vi "OCT ATS660.vi"() -> ()   [LabVIEW 2014]
doc: "I. Description:\nThis example demonstrates how to acquire a continuous amount of data (Waveform) using the DAQ device's internal clock.\n\nII. Instructions for Running:\n1. Create an analog input voltage channel.\n2. Set the rate for the sample clock. Additionally, define the sample mode to be continuous.\n3. Call the Start VI to start the acquisition.\n4. Read the waveform data in a loop until the user hits the stop button or an error occurs.\nNote: This example reads data from one or more channels and returns an array of data. Use the Index Array function to access an individual channel of data.\n5. Call the Clear Task VI to clear the Task.\n6. Use the popup dialog box to display an error if any.\n\nIV. I/O Connections Overview:\nMake sure your signal input terminal matches the Physical Channel I/O Control. For further connection information, refer to your hardware reference manual."
uses:
  Type Defs/OCT DAQ Channel Data Type.ctl
  Type Defs/Display States.ctl
  Saving Data/Saving Data States.ctl
  Type Defs/OCT Hardware States.ctl
  Type Defs/OCT Imaging Parameters Cluster.ctl
  Alazar VIs/ATS_ctl/ATS_Async_Setting.ctl
  Galvo VIs/galvo_states.ctl
  Alazar VIs/ATS_ctl/ATS_Global.ctl
  Alazar VIs/ATS_ctl/Record.ctl
  Alazar VIs/ATS_ctl/Clock.ctl
  Alazar VIs/ATS_ctl/ClockSource.ctl
  Alazar VIs/ATS_ctl/ClockRate.ctl
  Alazar VIs/ATS_ctl/ClockEdge.ctl
  Alazar VIs/ATS_ctl/InputCtrl.ctl
  Alazar VIs/ATS_ctl/Coupling.ctl
  Alazar VIs/ATS_ctl/Range.ctl
  Alazar VIs/ATS_ctl/Impedance.ctl
  Alazar VIs/ATS_ctl/Bandwidth.ctl
  Alazar VIs/ATS_ctl/Trigger.ctl
  Alazar VIs/ATS_ctl/TriggerOperation.ctl
  Alazar VIs/ATS_ctl/TriggerEngine.ctl
  Alazar VIs/ATS_ctl/ExtTrigger.ctl
  Alazar VIs/ATS_ctl/ExtTrigRange.ctl
  Signal Processing/processing_states.ctl
  En Face/En Face Depth Parameters.ctl
  Alazar VIs/ATS_ctl/ATS_Async_Ctrl.ctl
  Alazar VIs/ATS_ctl/ATS_Async_Mode.ctl
  Alazar VIs/ATS_ctl/ATS_DMA_Channel.ctl
  Alazar VIs/ATS_ctl/ATS_ReadSamples.ctl
  Alazar VIs/ATS_ctl/Device_Ctrl.ctl
  Alazar VIs/ATS_ctl/ATS_Check_Ctrl.ctl
  En Face/En Face States.ctl
  DAQ Status States.ctl
  Signal Processing/Display Raw Data states.ctl
panel:
  out "Background Array":u16[](array[numeric])
  in  "Calibrate":bool
  in  "Save Sweep Button":bool
  in  "Linear?":bool
  in  "Data Format":T1
  out "BScan":sgl[][](graph)
  in  "Display":T2
  in  "Save Sweep":bool
  in  "Stop Button":bool
  out "B-Scans Per Buffer":i32=1
  out "Current State":T3=enum."Aquire and Save"
  in  "Channels":tag="Dev2/ao0:1"
  in  "Trigger Source":tag="/Dev2/PFI7"
  in  "Imaging Parameters":T4={"Points Per A-Scan"=0, "A-Scans per B-Scan"=0, "Voltage Range"=1.0, "Card Resolution (bits)"=12}
  out "First Time?":bool=TRUE
  out "Save Data":bool
  in  "Async_Setting":T5
  out "Processing Finished":bool
  in  "OCT Hardware States":T3=enum."Acquire Clock"
  out "Save State":T6=enum."Do Nothing"
  out "Clock Length":u32=9184
  out "Reset DAQ":bool
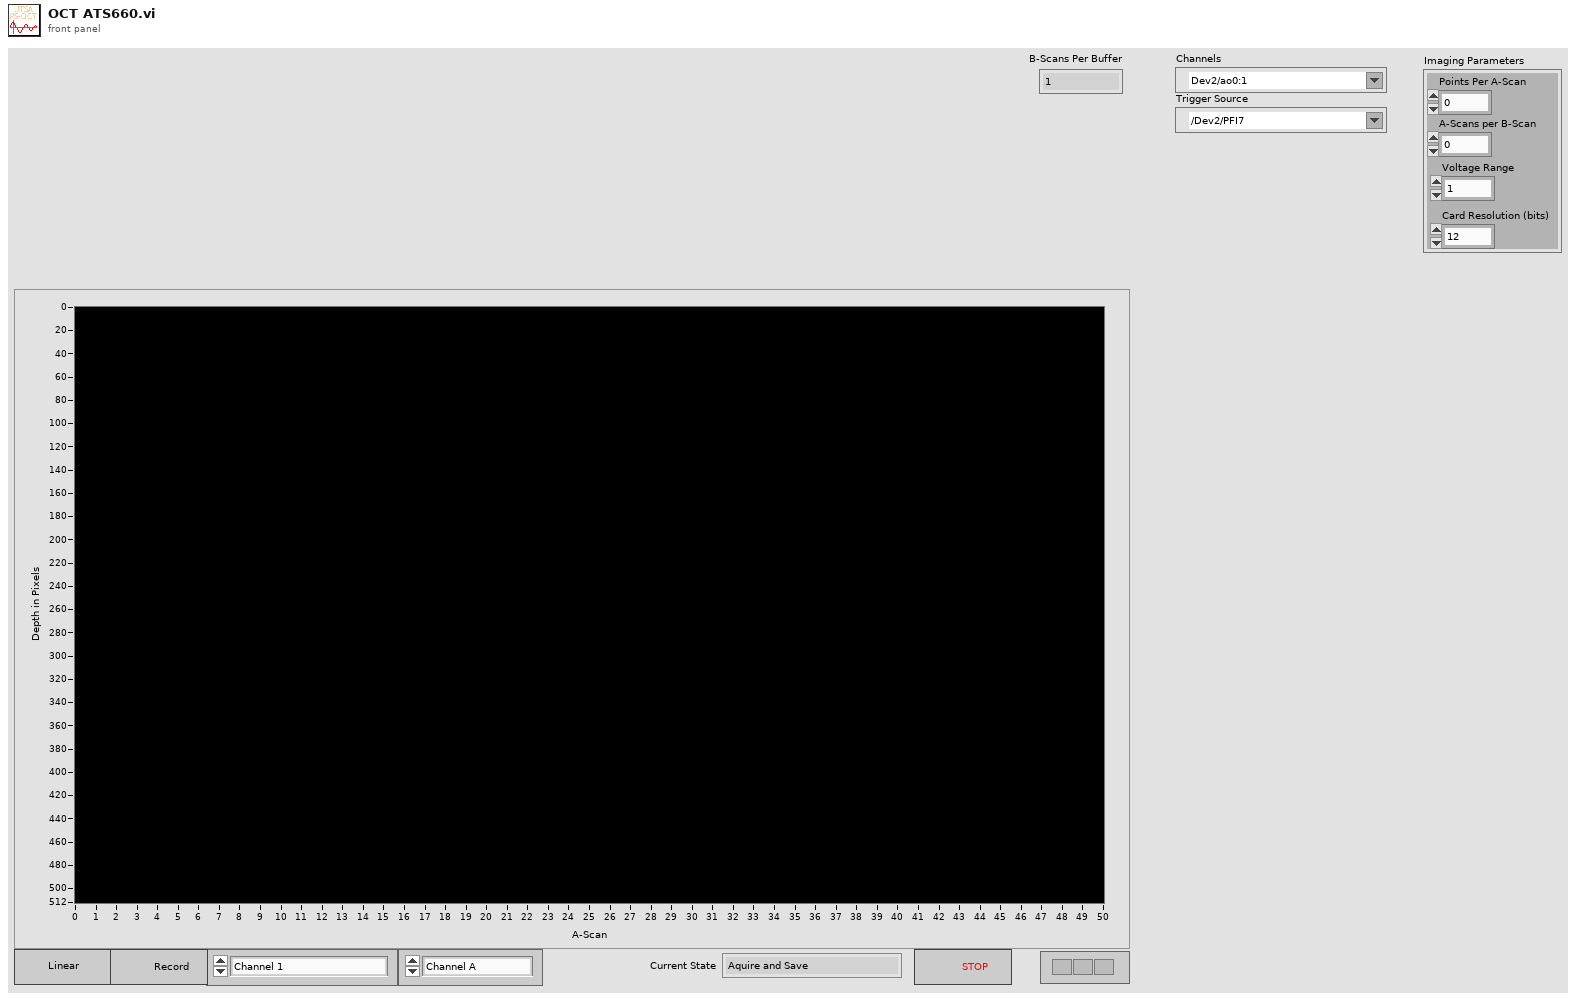
[diagram p1: front panel]
types:
  T1 = typedef "OCT DAQ Channel Data Type.ctl" = enum16{"Channel 1", "Channel 2", "Channel 1 and 2"}
  T2 = typedef "Display States.ctl" = enum16{"Channel A", "Channel B"}
  T3 = typedef "OCT Hardware States.ctl" = enum16{"Acquire Data", "Aquire and Save", "Allocate OpenCL Memory", "Delete OpenCL Memory", "Background Subtraction", "Acquire Background", "K-Space Calibration", "Update DAQ Parameters", "Initialize Clock", "Stop", "Wait", "Acquire Clock", "Initialize DAQ", "Set Resampling Array"}
  T4 = typedef "OCT Imaging Parameters Cluster.ctl" = cluster{"Points Per A-Scan":i32, "A-Scans per B-Scan":i32, "Voltage Range":sgl, "Card Resolution (bits)":u16}
  T5 = typedef "ATS_Async_Setting.ctl" = cluster{"UseHeader":u32, "Rec/Buffer":u32, "Total_Rec":u32, "DataBuffer":bool, "GetProcessedData":bool}
  T6 = typedef "Saving Data States.ctl" = enum16{"Get Queue Size", "Get Queue", "Get Timeout", "Flush Queue", "Close Files", "Create Files", "Do Nothing", "Initialize", "Enqueue Data", "Save Data", "Shutdown"}
  T7 = typedef "ATS_Global.ctl" = cluster{"Record":T8, "Clock":T9, "Input A":T13, "Input B":T13, "Trigger":T18}
  T8 = typedef "Record.ctl" = cluster{"Count":u32, "Presize":u32, "Length":u32}
  T9 = typedef "Clock.ctl" = cluster{"ClckSource":T10, "ClckRate":T11, "ClckEdge":T12, "Decimation":u32}
  T10 = typedef "ClockSource.ctl" = enum16{"Internal", "External", "Medium Ext.", "Slow Ext.", "Ext. AC", "Ext. DC", "Ext. (PLL)"}
  T11 = typedef "ClockRate.ctl" = u32
  T12 = typedef "ClockEdge.ctl" = u16
  T13 = typedef "InputCtrl.ctl" = cluster{"Coupling":T14, "Range":T15, "Impedance":T16, "Bandwidth":T17}
  T14 = typedef "Coupling.ctl" = enum16{"AC", "DC"}
  T15 = typedef "Range.ctl" = u32
  T16 = typedef "Impedance.ctl" = enum16{"1M ohms", "50 ohms"}
  T17 = typedef "Bandwidth.ctl" = enum16{"Full Bandwidth", "Reduce Bandwidth"}
  T18 = typedef "Trigger.ctl" = cluster{"TrigOperation":T19, "Timeout (s)":dbl, "Trig. Delay":u32, "Engine X":T20, "Engine Y":T20, "ExtTrigControl":T21}
  T19 = typedef "TriggerOperation.ctl" = enum16{"Only X", "Only Y", "X or Y", "X and Y", "X xor Y", "X and not Y", "not X and Y"}
  T20 = typedef "TriggerEngine.ctl" = cluster{"Source":enum32{"Chan_A", "Chan_B", "External", "Disable"}, "Slope":enum32{"Positive", "Negative"}, "Level":u32}
  T21 = typedef "ExtTrigger.ctl" = cluster{"Coupling":T14, "Range":T22}
  T22 = typedef "ExtTrigRange.ctl" = enum16{"1 V", "5 V", "TTL"}
  T23 = typedef "galvo_states.ctl" = enum16{"Reset", "Reset Galvos?", "Center Galvos", "Register Callback", "Get Scan Parameters", "Show", "Initialize", "Run Raster", "Load Raster", "Run Circle", "Shutdown"}
  T24 = typedef "processing_states.ctl" = enum16{"Initialize", "Set Background", "Update Imaging Parameters", "Get Queue", "Process Data", "Get Size", "Flush Data", "Set Reample Array", "Get Last Processed BScan", "Shutdown"}
  T25 = typedef "En Face Depth Parameters.ctl" = cluster{"En Face Start\nDepth":i32, "En Face End\nDepth":i32}
  T26 = typedef "En Face States.ctl" = enum16{"Save BMP", "Show", "Clear En Face", "Update EnFace"}
  T27 = typedef "Scanning Cluster.ctl" = cluster{"Fast Axis Offset":sgl, "Slow Axis Offset":sgl, "Slow Axis Amp":sgl, "Fast Axis Amp":sgl, "B-scans (rings)":u32, "A(cluster)/B":u32, "Scan Pattern":enum16{"Raster"}}
  T28 = typedef "Processed OCT Data.ctl" = cluster{"Intensity A":sgl[][][], "Intensity B":sgl[][][]}
  T29 = typedef "ATS_Async_Ctrl.ctl" = enum16{"SetupDMA", "StartCapture", "Get", "Get_Stream", "Abort", "Stop"}
  T30 = typedef "ATS_ReadSamples.ctl" = cluster{"Offset":i32, "Length":u32}
  T31 = typedef "ATS_DMA_Channel.ctl" = enum16{"Channel_A", "Channel_B", "A & B"}
  T32 = typedef "ATS_Async_Mode.ctl" = enum16{"Continuous", "Triggered", "No-Pre-Trigger", "Traditional"}
  T33 = typedef "ATS_Check_Ctrl.ctl" = enum16{"None", "NO_ATS9462", "ATS9462_Traditional", "Verify Board", "OnBoard Memory", "Board & Memory", "Master/Slave", "NO Master/Slave"}
  T34 = typedef "Device_Ctrl.ctl" = enum16{"Status", "About", "Arm", "ForceTrig", "Abort", "Initialize", "Init (NoPreset)", "Info", "Close", "Calibrate", "SetManually", "LED_ON", "LED_OFF"}
  T35 = typedef "DAQ Status States.ctl" = enum16{"Get", "Show"}
  T36 = typedef "ATS_Async_Status.ctl" = cluster{"Start DMA":bool, "StartCapture":bool, "Valid":bool, "Completed":bool, "InProgress":bool, "Timeout":bool, "Overflow":bool, "Error":bool}
  T37 = typedef "Display Raw Data states.ctl" = enum16{"Add Raw", "Add Processed", "Show"}
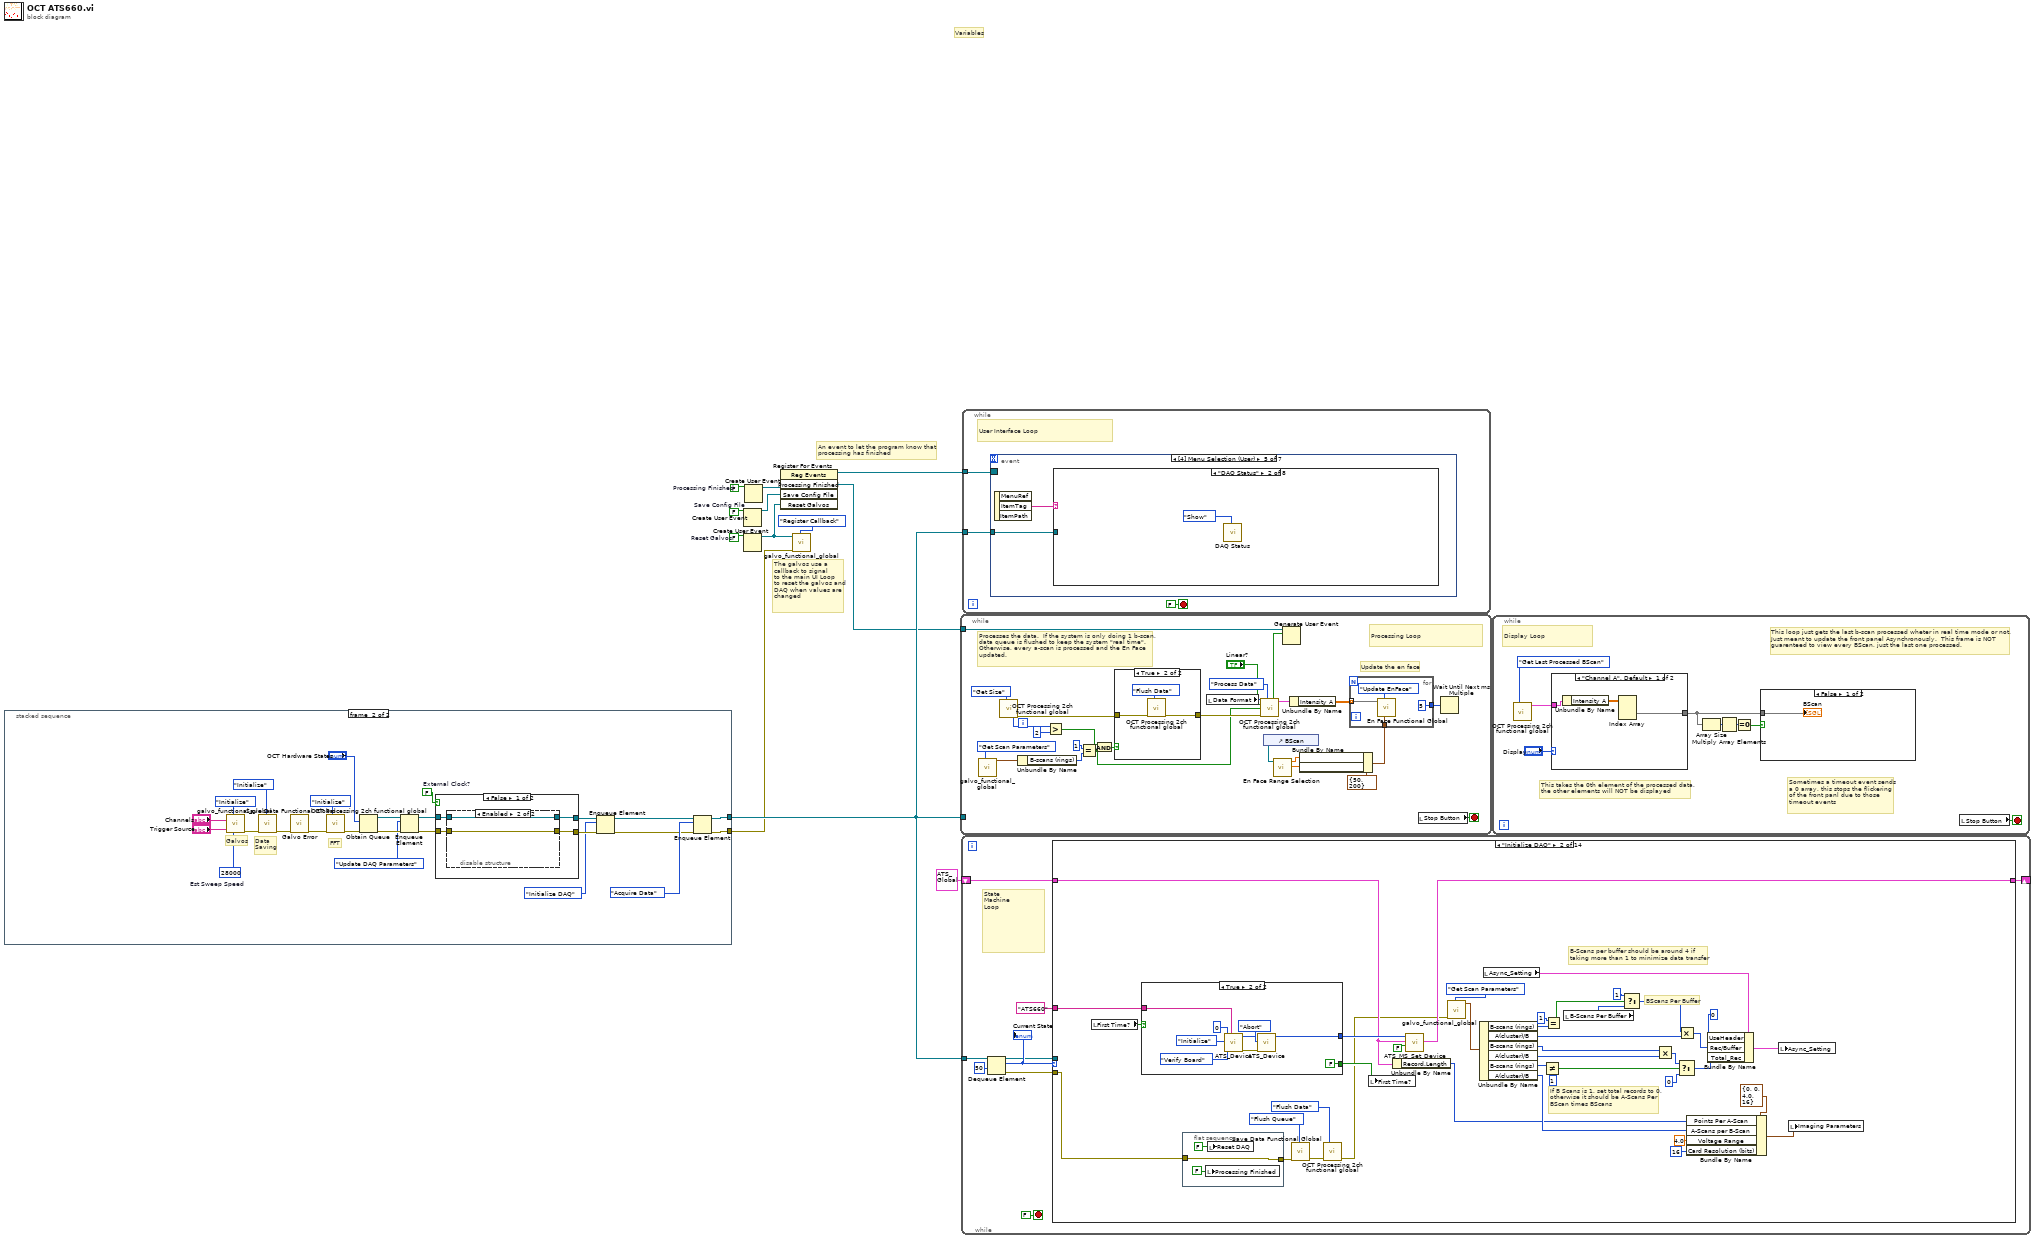
[diagram p0: block diagram]
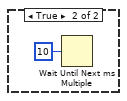
[diagram p3: hidden frame]
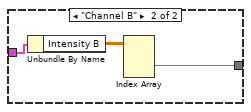
[diagram p4: hidden frame]
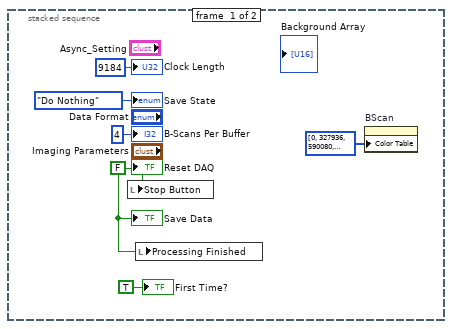
[diagram p5: hidden frame]
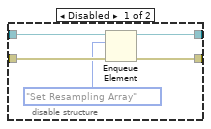
[diagram p6: hidden frame]
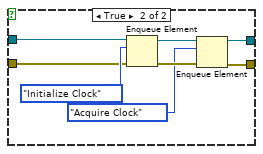
[diagram p7: hidden frame]
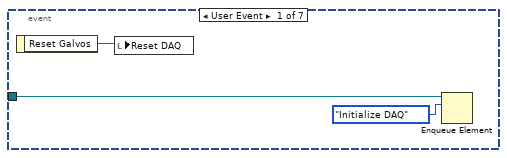
[diagram p8: hidden frame]
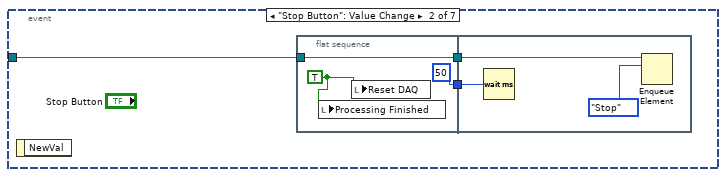
[diagram p9: hidden frame]
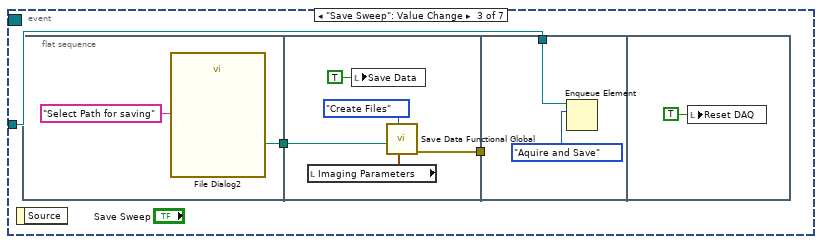
[diagram p10: hidden frame]
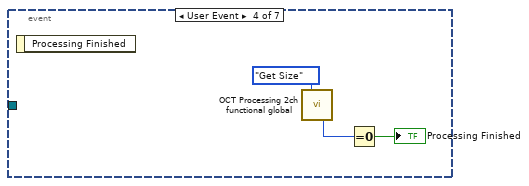
[diagram p11: hidden frame]
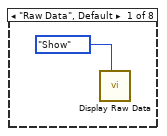
[diagram p12: hidden frame]
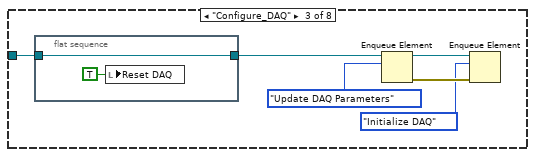
[diagram p13: hidden frame]
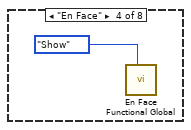
[diagram p14: hidden frame]
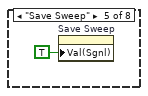
[diagram p15: hidden frame]
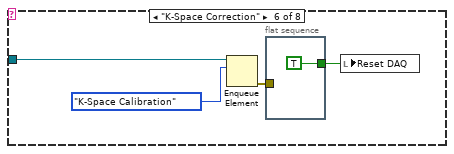
[diagram p16: hidden frame]
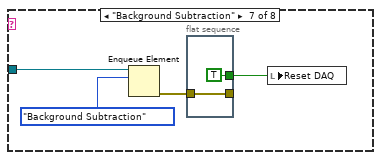
[diagram p17: hidden frame]
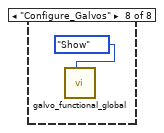
[diagram p18: hidden frame]
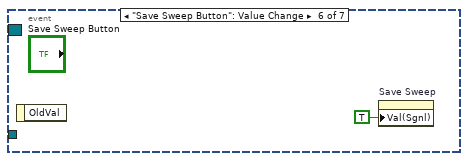
[diagram p19: hidden frame]
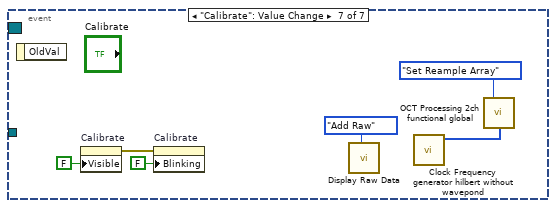
[diagram p20: hidden frame]
diagram:
  w5 = FALSE  # Reset Galvos
  w8 = FALSE  # Save Config File
  w11 = FALSE  # Processing Finished
  # "The galvos use a \ncallback to signal\nto the main UI Loop\nto reset the galvos and\nDAQ when values are\nchanged"
  # "An event to let the program know that\nprocessing has finished"
  # "Variables"
  n1 = stacked-sequence {
    tunnel: [_ w26] -> w9
    tunnel: [_ w25] -> w1
    frame #0 {
      w14 = FALSE ("Sweep Ready for saving")
      n2 = local write "Stop Button"(w14) -> ()
      n3 = local write "Processing Finished"(w14) -> ()
      n4 = property on="BScan" class="IntGraph (strict)"("Color Table"=u32[] [0, 327936, 590080, 852224, 983296, 1114624, 1180160, 1311232, 1442304, 1573632, 1704704, 1770240, 1901312, 1966848, 2098176, 2163712, 2294784, 2491392, 2557184, 2688256, 2753792, 2884864, 2950656, 3081728, 3147264, 3344129, 3475457, 3540993, 3672321, 3738113, 3869185, 3934977, 4066305, 4197633, 4328961, 4394497, 4460289, 4591617, 4657409, 4788481, 4854273, 4985601, 5116929, 5248257, 5314049, 5379841, 5511169, 5576961, 5708033, 5773825, 5905153, 6036482, 6167810, 6233346, 6299138, 6430466, 6496258, 6562050, 6693634, 6759426, 6890754, 7022082, 7087874, 7153666, 7284994, 7350786, 7482114, 7547906, 7613698, 7745026, 7876354, 8007682, 8073474, 8139522, 8205314, 8336642, 8467970, 8533763, 8599555, 8665347, 8731139, 8862467, 8993795, 9059587, 9125380, 9191428, 9257220, 9388548, 9454340, 9520132, 9585924, 9717253, 9848837, 9914629, 9980165, 10045957, 10177541, 10243334, 10309126, 10375174, 10440966, 10572294, 10703623, 10769416, 10835208, 10901256, 10967049, 11033097, 11033609, 11099401, 11165450, 11231242, 11231754, 11297547, 11363339, 11429131, 11495180, 11495692, 11561740, 11693069, 11758861, 11759373, 11825165, 11891214, 11957006, 12022799, 12023311, 12089103, 12220944, 12286736, 12286736, 12352529, 12418577, 12484370, 12550162, 12615954, 12681747, 12747796, 12813588, 12813845, 12879894, 12945686, 13077015, 13142808, 13143064, 13208856, 13274905, 13340697, 13340953, 13472282, 13538075, 13604379, 13670172, 13735964, 13801757, 13867550, 13933343, 13999392, 13999648, 14065441, 14131234, 14197027, 14197541, 14263334, 14329383, 14395176, 14460969, 14592553, 14658346, 14724139, 14789932, 14790189, 14856238, 14922287, 14988080, 15053873, 15054130, 15119923, 15185972, 15251765, 15317559, 15383353, 15449146, 15449660, 15515454, 15515968, 15516226, 15582021, 15582278, 15582536, 15648587, 15648844, 15714639, 15714897, 15715155, 15780949, 15781463, 15847256, 15847770, 15848028, 15913823, 15914081, 15979875, 15980133, 15980391, 16046441, 16046444, 16046703, 16046705, 16112500, 16113015, 16113274, 16113277, 16179072, 16179330, 16179588, 16245384, 16245387, 16245389, 16245648, 16311443, 16376982, 16377241, 16377499, 16443294, 16443553, 16443555, 16443815, 16509866, 16510124, 16510127, 16575923, 16575924, 16576182, 16576441, 16576443, 16576702, 16576705, 16576963, 16577222, 16577224, 16577482, 16577485, 16577743, 16577745, 16578004, 16578262, 16578264, 16578523, 16578782, 16579040, 16579299, 16579301, 16579303, 16579562, 16579821]) -> ()  [unwired: 2 in, 2 out]
      "B-Scans Per Buffer" <- 4 ("B-Scans Per Buffer")
      "Clock Length" <- u32 9184 ("Clock Length")
      "Save State" <- Saving_Data_States."Do Nothing" ("Save State")
      "Reset DAQ" <- w14
      "Save Data" <- w14
      "First Time?" <- TRUE ("First Time?")
    }
    frame #1 {
      w30 = 28000  # Est Sweep Speed
      w31 = FALSE  # External Clock?
      # "FFT"
      # "Data \nSaving"
      # "Galvos"
      n5 = call "galvo_functional_global.vi"("Est Sweep Speed"=w30, "State"=galvo_states."Initialize", "Trigger Source"="Trigger Source", "Analog Output"="Channels") -> ("error out"=w35:errorcluster)  [unwired: 6 in, 1 out]
      n6 = call "Save Data Functional Global.vi"("States"=Saving_Data_States."Initialize", "error in (no error)"=w35) -> ("error out"=w21:errorcluster)  [unwired: 6 in, 3 out]
      n7 = call "Galvo Error.vi"("error in (no error)"=w21) -> ("error out"=w20:errorcluster)  [unwired: 10 in]
      n8 = call "OCT Processing 2ch functional global.vi"("State"=processing_states."Initialize", "error in (no error)"=w20) -> ("error out"=w38:errorcluster)  [unwired: 9 in, 4 out]
      n9 = Obtain Queue(element data type="OCT Hardware States", error in (no error)=w38) -> (queue out=w28:refnum<queue>, error out=w29:errorcluster)  [unwired: 3 in, 1 out]
      n10 = Enqueue Element(queue=w28, element=OCT_Hardware_States."Update DAQ Parameters", error in (no error)=w29) -> (queue out=w23:refnum<queue>, error out=w22:errorcluster)  [unwired: 1 in, 1 out]
      n11 = case shown="False" w31 {
        tunnel: [w43 w59] -> w42
        tunnel: [w44 w58] -> w41
        tunnel: w23 -> [w46 w55]
        tunnel: w22 -> [w45 w54]
        frame False {
          n12 = disable-structure shown="Enabled" {
            disable-tunnel: w46 -> [w51 w53]
            disable-tunnel: w45 -> [w50 w52]
            disable-tunnel: [w49 w52] -> w44
            disable-tunnel: [w48 w53] -> w43
            frame Disabled {
              n13 = Enqueue Element(queue=w51, element=OCT_Hardware_States."Set Resampling Array", error in (no error)=w50) -> (queue out=w48:refnum<queue>, error out=w49:errorcluster)  [unwired: 1 in, 1 out]
            }
            frame Enabled {
            }
          }
        }
        frame True {
          n14 = Enqueue Element(queue=w55, element=OCT_Hardware_States."Initialize Clock", error in (no error)=w54) -> (queue out=w61:refnum<queue>, error out=w60:errorcluster)  [unwired: 1 in, 1 out]
          n15 = Enqueue Element(queue=w61, element=OCT_Hardware_States."Acquire Clock", error in (no error)=w60) -> (queue out=w59:refnum<queue>, error out=w58:errorcluster)  [unwired: 1 in, 1 out]
        }
      }
      n16 = Enqueue Element(queue=w42, element=OCT_Hardware_States."Initialize DAQ", error in (no error)=w41) -> (queue out=w18:refnum<queue>, error out=w19:errorcluster)  [unwired: 1 in, 1 out]
      n17 = Enqueue Element(queue=w18, element=OCT_Hardware_States."Acquire Data", error in (no error)=w19) -> (queue out=w26:refnum<queue>, error out=w25:errorcluster)  [unwired: 1 in, 1 out]
    }
  }
  n18 = Create User Event(user event datatype=w8) -> (user event=w7:refnum<user-event>)  [unwired: 1 in, 1 out]
  n19 = Create User Event(user event datatype=w5) -> (user event=w4:refnum<user-event>)  [unwired: 1 in, 1 out]
  n20 = Create User Event(user event datatype=w11) -> (user event=w6:refnum<user-event>)  [unwired: 1 in, 1 out]
  n21 = register-events(w6, w7, w4) -> (reference out=w10:refnum<event-registration>)  [unwired: 2 in, 1 out]
  n22 = call "galvo_functional_global.vi"("State"=galvo_states."Register Callback", "error in (no error)"=w1, "user event out"=w4) -> ()  [unwired: 7 in, 2 out]
  n23 = while {
    tunnel: w6 -> [w77]
    tunnel: w9 -> [_]
    stop <- w87 stop-if-true
    # "Processing Loop"
    # "Update the en face"
    # "Processes the data.  If the system is only doing 1 b-scan, \ndata queue is flushed to keep the system \"real time\".\nOtherwise, every a-scan is processed and the En Face\nupdated."
    n24 = call "galvo_functional_global.vi"("State"=galvo_states."Get Scan Parameters") -> ("Scanning Output"=w71:T27)  [unwired: 9 in, 1 out]
    n25 = call "OCT Processing 2ch functional global.vi"("State"=processing_states."Get Size") -> ("# elements in queue"=w83:i32, "error out"=w74:errorcluster)  [unwired: 10 in, 3 out]
    n26 = Unbundle By Name(w71) -> ("B-scans (rings)"=w79:u32)
    n27 = Greater?(x=w83, y=2) -> (0:w84:bool)
    n28 = Equal?(x=u32 1, y=w79) -> (x = y?=w67:bool)
    n29 = And(x=w84, y=w67) -> (x .and. y?=w72:bool)
    n30 = case shown="True" w72 {
      tunnel: w74 -> [w92 w95]
      tunnel: [w92 w94] -> w73
      frame False {
      }
      frame True {
        n31 = call "OCT Processing 2ch functional global.vi"("State"=processing_states."Flush Data", "error in (no error)"=w95) -> ("error out"=w94:errorcluster)  [unwired: 9 in, 4 out]
      }
    }
    n32 = local read "Data Format"() -> (w78:T1)
    n33 = call "OCT Processing 2ch functional global.vi"("Data Format"=w78, "State"=processing_states."Process Data", "Linear?"="Linear?", "Real Time"=w67, "error in (no error)"=w73) -> ("Time Out"=w76:bool, "Processed OCT Data"=w81:T28)  [unwired: 6 in, 3 out]
    n34 = control-ref of="BScan"() -> (w66:refnum<vi>)
    n35 = call "En Face Range Selection.vi"("IntensityGraph in"=w66) -> ("Lower En Face"=w63:dbl, "Upper En Face"=w64:dbl)  [unwired: 9 in]
    n36 = Generate User Event(user event=w77, event data cluster=w76) -> ()  [unwired: 2 in, 2 out]
    n37 = Unbundle By Name(w81) -> ("Intensity A"=w75:sgl[][][])
    n38 = Bundle By Name(cluster=T25 {"En Face Start\nDepth"=50, "En Face End\nDepth"=200} ("En Face Parameters"), "En Face Start\nDepth"=w64, "En Face End\nDepth"=w63) -> (w62:T25)
    n39 = for {
      tunnel: w75 -> [w90] mode=indexing
      tunnel: [u32 5 ("millisecond multiple")] -> w69
      tunnel: w62 -> [w88]
      n40 = call "En Face Functional Global.vi"("En Face Parameters"=w88, "En Face States"=En_Face_States."Update EnFace", "B Scan In"=w90) -> ()  [unwired: 8 in, 1 out]
    }
    n41 = local read "Stop Button"() -> (w87:bool)
    n42 = Wait Until Next ms Multiple(millisecond multiple=w69) -> ()  [unwired: 1 out]
  }
  n43 = while {
    tunnel: w9 -> [w104]
    shift-right: [w98] -> _
    shift-left: T7 {"Record"={"Count"=0, "Presize"=0, "Length"=0}, "Clock"={"ClckSource"=enum."Internal", "ClckRate"=0, "ClckEdge"=0, "Decimation"=0}, "Input A"={"Coupling"=enum."DC", "Range"=12, "Impedance"=enum."1M ohms", "Bandwidth"=enum."Full Bandwidth"}, "Input B"={"Coupling"=enum."DC", "Range"=12, "Impedance"=enum."1M ohms", "Bandwidth"=enum."Full Bandwidth"}, "Trigger"={"TrigOperation"=enum."Only X", "Timeout (s)"=-1.0, "Trig. Delay"=0, "Engine X"={"Source"=enum."Chan_A", "Slope"=enum."Positive", "Level"=0}, "Engine Y"={"Source"=enum."Chan_A", "Slope"=enum."Positive", "Level"=0}, "ExtTrigControl"={"Coupling"=enum."AC", "Range"=enum."1 V"}}} ("Value") -> [w97]
    stop <- FALSE stop-if-true
    # "State\nMachine\nLoop"
    n44 = Dequeue Element(queue=w104, timeout in ms (-1)=50) -> (queue out=w100:refnum<queue>, element=w102:T3, error out=w101:errorcluster)  [unwired: 1 in, 1 out]
    "Current State" <- w102
    n45 = case shown="\"Initialize DAQ\"" w102 {
      tunnel: w101 -> [_ w148 w205 w257 w311 _ w369 _ _ _ w407 w415 _ _]
      tunnel: w100 -> [_ _ w206 w256 w325 _ w370 _ _ _ w408 w413 _ _]
      tunnel: "ATS660" ("BoardToVerify") -> [_ w162 _ _ _ _ _ w377 _ w393 _ _ _ _]
      tunnel: [w121 w156 w222 w268 w300 w359 w361 w376 w392 w394 w403 w417 w420 w421] -> w98
      tunnel: w97 -> [w121 w155 w222 w268 w300 w359 w361 w376 w392 _ w403 w417 w420 w421]
      frame "Acquire Clock" {
        w108 = 0 ("DeviceIn")
        n46 = local read "Clock Length"() -> (w110:u32)
        n47 = local read "Async_Setting"() -> (w106:T5)
        n48 = Bundle By Name(cluster=w106, "UseHeader"=u32 0, "Rec/Buffer"=u32 125, "Total_Rec"=u32 0) -> (w107:T5)
        n49 = Unbundle By Name(w121) -> ("Record.Presize"=w111:u32)
        n50 = Bundle By Name(cluster=T30 {"Offset"=0, "Length"=0} ("ReadSamples"), "Length"=w110, "Offset"=w111) -> (w109:T30)
        n51 = call "ATS_AsyncDMA_Device.vi"("DeviceIn"=w108, "ATS_Async_Ctrl"=ATS_Async_Ctrl."SetupDMA" ("ATS_DMA_Ctrl"), "Async_Mode"=ATS_Async_Mode."Traditional", "Async_Setting"=w107, "Channel"=ATS_DMA_Channel."Channel_B", "ReadSamples"=w109, "Start Now / Wait"=TRUE) -> ("Buffer"=w116:u16[])  [unwired: 4 in, 4 out]
        n52 = while {
          tunnel: w116 -> [_]
          shift-right: [ATS_Async_Ctrl."Get" ("ATS_Async_Ctrl")] -> _
          shift-left: ATS_Async_Ctrl."StartCapture" ("ATS_Async_Ctrl") -> [w130]
          tunnel: w108 -> [w125]
          stop <- w128 stop-if-true
          n53 = call "ATS_AsyncDMA_Device.vi"("DeviceIn"=w125, "ATS_Async_Ctrl"=w130) -> ("Buffer"=w123:u16[], "Async_Status"=w122:T36)  [unwired: 9 in, 3 out]
          n54 = Unbundle By Name(w122) -> ("Valid"=w124:bool, "Completed"=w132:bool, "Start DMA"=w133:bool, "Timeout"=w134:bool, "Error"=w131:bool)
          n55 = local read "Clock Length"() -> (w126:u32)
          n56 = Compound Arithmetic op=OR(w132, invert w133, w134, w131) -> (w127:bool)
          n57 = case shown="False" w124 {
            selector: w124 -> [w135 w138]
            tunnel: w123 -> [_ w137]
            tunnel: [w135 w138] -> w128
            tunnel: w127 -> [_ _]
            tunnel: w126 -> [_ w136]
            frame False {
            }
            frame True {
              n58 = Array Subset(array=w137, length=w136) -> (w139:u16[])  [unwired: 1 in]
              n59 = call "Clock Frequency generator hilbert.vi"("End of clock"=6300.0 ("Sweep Speed"), "Acquisition speed (S/s)"=180000000.0 ("Sweep Speed"), "k-space signal in"=w139, "number of frequency updates"=4385) -> ("Error Out"=w144:errorcluster, "frequency\nsteps"=w143:i32)  [unwired: 6 in]
              n60 = call "wavepond sequence.vi"("Error In"=w144, "Number of updates"=w143) -> ()  [unwired: 9 in, 1 out]
            }
          }
        }
      }
      frame "Initialize DAQ" {
        # "B-Scans per buffer should be around 4 if \ntaking more than 1 to minimize data transfer"
        # "If B Scans is 1, set total records to 0,\notherwise it should be A-Scans Per\nBScan times BScans"
        # "BScans Per Buffer"
        n61 = local read "First Time?"() -> (w159:bool)
        n62 = case shown="True" w159 {
          tunnel: [w188 w198] -> w184
          tunnel: w162 -> [_ w194]
          tunnel: [FALSE ("First Time?") FALSE ("First Time?")] -> w158
          frame False {
            n63 = flat-sequence {
              tunnel: [w190] -> w188
              frame #0 {
                w190 = 0 ("DeviceIn")
                n64 = call "ATS_AsyncDMA_Device.vi"("DeviceIn"=w190, "ATS_Async_Ctrl"=ATS_Async_Ctrl."Stop") -> ("ReadSamples_Out"=w193:T30)  [unwired: 9 in, 4 out]
                n65 = call "ATS_AsyncDMA_Device.vi"("DeviceIn"=w190, "ATS_Async_Ctrl"=ATS_Async_Ctrl."Abort", "ReadSamples"=w193) -> ()  [unwired: 8 in, 5 out]
              }
            }
          }
          frame True {
            n66 = call "ATS_Device.vi"("BoardToVerify"=w194, "ATS_Check"=ATS_Check_Ctrl."Verify Board", "DevCtrl"=Device_Ctrl."Initialize", "DeviceIn"=0 ("Device")) -> ("error out"=w196:errorcluster, "DeviceOut"=w200:i32)  [unwired: 1 in, 5 out]
            n67 = call "ATS_Device.vi"("error in (no error)"=w196, "DevCtrl"=Device_Ctrl."Abort", "DeviceIn"=w200) -> ("DeviceOut"=w198:i32)  [unwired: 2 in, 6 out]
          }
        }
        n68 = flat-sequence {
          tunnel: w148 -> [w186]
          tunnel: [w186] -> w149
          frame #0 {
            n69 = local write "Processing Finished"(FALSE ("Reset DAQ")) -> ()
            n70 = local write "Reset DAQ"(FALSE ("Reset DAQ")) -> ()
          }
        }
        n71 = call "Save Data Functional Global.vi"("States"=Saving_Data_States."Flush Queue", "error in (no error)"=w149) -> ("error out"=w151:errorcluster)  [unwired: 6 in, 3 out]
        n72 = call "OCT Processing 2ch functional global.vi"("State"=processing_states."Flush Data", "error in (no error)"=w151) -> ("error out"=w147:errorcluster)  [unwired: 9 in, 4 out]
        n73 = local write "First Time?"(w158) -> ()
        n74 = Unbundle By Name(w155) -> ("Record.Length"=w163:u32)
        n75 = call "ATS_MS_Set_Device.vi"("Set_Manually (F)"=FALSE, "Setup_In"=w155, "DeviceIn"=w184) -> ("Setup_Out"=w156:T7)  [unwired: 3 in, 5 out]
        n76 = call "galvo_functional_global.vi"("State"=galvo_states."Get Scan Parameters", "error in (no error)"=w147) -> ("Scanning Output"=w154:T27)  [unwired: 8 in, 1 out]
        n77 = Unbundle By Name(w154) -> ("B-scans (rings)"=w169:u32, "A(cluster)/B"=w179:u32, "B-scans (rings)"=w174:u32, "A(cluster)/B"=w173:u32, "B-scans (rings)"=w171:u32, "A(cluster)/B"=w165:u32)
        n78 = local read "Async_Setting"() -> (w161:T5)
        n79 = Not Equal?(x=w171, y=u32 1 ("x")) -> (x != y?=w172:bool)
        n80 = Equal?(x=u32 1, y=w169) -> (x = y?=w175:bool)
        n81 = local read "B-Scans Per Buffer"() -> (w157:i32)
        n82 = Select(t=u32 1 ("y"), s=w175, f=w157) -> (s? t:f=w177:u32)
        n83 = Multiply(x=w174, y=w173) -> (x*y=w168:u32)
        n84 = Select(t=w168, s=w172, f=u32 0 ("Total_Rec")) -> (s? t:f=w182:u32)
        n85 = Multiply(x=w177, y=w179) -> (x*y=w180:u32)
        n86 = Bundle By Name(cluster=T4 {"Points Per A-Scan"=0, "A-Scans per B-Scan"=0, "Voltage Range"=4.0, "Card Resolution (bits)"=16} ("Imaging Parameters"), "Points Per A-Scan"=w163, "A-Scans per B-Scan"=w165, "Voltage Range"=sgl 4.0, "Card Resolution (bits)"=u16 16) -> (w164:T4)
        n87 = Bundle By Name(cluster=w161, "UseHeader"=u32 0, "Rec/Buffer"=w180, "Total_Rec"=w182) -> (w160:T5)
        n88 = local write "Async_Setting"(w160) -> ()
        n89 = local write "Imaging Parameters"(w164) -> ()
      }
      frame "Acquire Data", Default {
        # "Update and \nclear the \nEn Face"
        # "Tell the FFT the most\nup-to-date imaging\nparameters"
        n90 = Enqueue Element(queue=w206, element=OCT_Hardware_States."Initialize DAQ", error in (no error)=w205) -> (error out=w203:errorcluster)  [unwired: 1 in, 2 out]
        n91 = local read "Imaging Parameters"() -> (w227:T4)
        n92 = call "galvo_functional_global.vi"("State"=galvo_states."Run Raster", "error in (no error)"=w203) -> ("error out"=w218:errorcluster)  [unwired: 8 in, 1 out]
        n93 = local read "Async_Setting"() -> (w226:T5)
        n94 = call <vilib>:"Clear Errors.vi"("error in (no error)"=w218) -> ("error out"=w217:errorcluster)  [unwired: 5 in, 1 out]
        n95 = call "OCT Processing 2ch functional global.vi"("State"=processing_states."Update Imaging Parameters", "Input Parameters"=w227, "error in (no error)"=w217) -> ("error out"=w210:errorcluster)  [unwired: 8 in, 4 out]
        n96 = local read "Data Format"() -> (w229:T1)
        n97 = call "galvo_functional_global.vi"("State"=galvo_states."Get Scan Parameters", "error in (no error)"=w210) -> ("error out"=w211:errorcluster, "Scanning Output"=w219:T27)  [unwired: 8 in]
        n98 = call "Quick NPT Config.vi"("error in (no error)"=w203, "Data Format"=w229, "Async_Setting"=w226, "Value"=w222) -> ("error out"=w207:errorcluster, "Device Out"=w232:i32, "Record Length"=w212:u32)  [unwired: 4 in]
        n99 = call "En Face Functional Global.vi"("En Face States"=En_Face_States."Clear En Face", "Error In"=w211, "Scanning"=w219) -> ("Error Out"=w209:errorcluster)  [unwired: 8 in]
        n100 = Merge Errors(w207, w209) -> (w208:errorcluster)
        n101 = call "OCT Processing 2ch functional global.vi"("State"=processing_states."Get Queue", "error in (no error)"=w208) -> ("queue out"=w224:refnum<queue>, "error out"=w216:errorcluster)  [unwired: 9 in, 3 out]
        n102 = while {
          tunnel: w232 -> [w252]
          shift-right: [ATS_Async_Ctrl."Get" ("ATS_Async_Ctrl")] -> _
          shift-left: ATS_Async_Ctrl."StartCapture" ("ATS_Async_Ctrl") -> [w251]
          tunnel: w224 -> [w247]
          tunnel: [w246] -> w223
          tunnel: w212 -> [w245]
          tunnel: w216 -> [w241]
          tunnel: [w241] -> w215
          stop <- w246 stop-if-true
          n103 = call "ATS_AsyncDMA_Device.vi"("DeviceIn"=w252, "ATS_Async_Ctrl"=w251) -> ("Buffer"=w249:u16[], "Async_Status"=w244:T36)  [unwired: 9 in, 3 out]
          n104 = local read "Reset DAQ"() -> (w248:bool)
          n105 = call "DAQ Status.vi"("Enum"=DAQ_Status_States."Get", "Async_Status"=w244) -> ("DAQ Error?"=w242:bool, "Valid"=w243:bool)  [unwired: 8 in]
          n106 = Compound Arithmetic op=OR(w242, w248) -> (w246:bool)
          n107 = case shown="True" w243 {
            tunnel: w249 -> [_ w253]
            tunnel: w247 -> [_ w255]
            tunnel: w245 -> [_ _]
            frame False {
              # "Do nothing"
            }
            frame True {
              n108 = Enqueue Element(queue=w255, element=w253, timeout in ms (-1)=50) -> ()  [unwired: 1 in, 3 out]
            }
          }
        }
        n109 = while {
          tunnel: w223 -> [w239]
          tunnel: [w236] -> w214
          tunnel: w215 -> [w236]
          stop <- w233 stop-if-true
          n110 = local read "Processing Finished"() -> (w238:bool)
          n111 = Wait (ms)(milliseconds to wait=u32 25) -> ()  [unwired: 1 out]
          n112 = local read "Reset DAQ"() -> (w234:bool)
          n113 = And(x=w239, y=w238) -> (x .and. y?=w235:bool)
          n114 = Or(x=w235, y=w234) -> (x .or. y?=w233:bool)
        }
        n115 = call "galvo_functional_global.vi"("State"=galvo_states."Reset", "error in (no error)"=w214) -> ()  [unwired: 8 in, 2 out]
      }
      frame "Acquire Background" {
        # "Update and \nclear the \nEn Face"
        # "Tell the FFT the most\nup-to-date imaging\nparameters"
        n116 = local read "Imaging Parameters"() -> (w270:T4)
        n117 = call "galvo_functional_global.vi"("State"=galvo_states."Run Raster", "error in (no error)"=w257) -> ("error out"=w265:errorcluster)  [unwired: 8 in, 1 out]
        n118 = local read "Async_Setting"() -> (w269:T5)
        n119 = call <vilib>:"Clear Errors.vi"("error in (no error)"=w265) -> ("error out"=w264:errorcluster)  [unwired: 5 in, 1 out]
        n120 = call "OCT Processing 2ch functional global.vi"("State"=processing_states."Update Imaging Parameters", "Input Parameters"=w270, "error in (no error)"=w264) -> ("error out"=w263:errorcluster)  [unwired: 8 in, 4 out]
        n121 = local read "Data Format"() -> (w271:T1)
        n122 = call "galvo_functional_global.vi"("State"=galvo_states."Get Scan Parameters", "error in (no error)"=w263) -> ("error out"=w261:errorcluster)  [unwired: 8 in, 1 out]
        n123 = call "Quick NPT Config.vi"("error in (no error)"=w257, "Data Format"=w271, "Async_Setting"=w269, "Value"=w268) -> ("error out"=w262:errorcluster, "Device Out"=w274:i32)  [unwired: 4 in, 1 out]
        n124 = Merge Errors(w262, w261) -> (w258:errorcluster)
        n125 = while {
          tunnel: w274 -> [w284]
          shift-right: [ATS_Async_Ctrl."Get" ("ATS_Async_Ctrl")] -> _
          shift-left: ATS_Async_Ctrl."StartCapture" ("ATS_Async_Ctrl") -> [w283]
          tunnel: w258 -> [w280]
          tunnel: [w280] -> w259
          stop <- w276 stop-if-true
          n126 = local read "Imaging Parameters"() -> (w277:T4)
          n127 = call "ATS_AsyncDMA_Device.vi"("DeviceIn"=w284, "ATS_Async_Ctrl"=w283) -> ("Buffer"=w278:u16[], "Async_Status"=w281:T36)  [unwired: 9 in, 3 out]
          n128 = call "DAQ Status.vi"("Enum"=DAQ_Status_States."Get", "Async_Status"=w281) -> ("Valid"=w279:bool)  [unwired: 8 in, 1 out]
          n129 = case shown="True" w279 {
            selector: w279 -> [_ w289]
            tunnel: w278 -> [_ w293]
            tunnel: w277 -> [_ w292]
            tunnel: [FALSE w289] -> w276
            frame False {
            }
            frame True {
              n130 = Unbundle By Name(w292) -> ("A-Scans per B-Scan"=w291:i32, "Points Per A-Scan"=w290:i32)
              n131 = Reshape Array(w293, w291, w290) -> (w287:u16[][])
              n132 = call "Average BScan.vi"("B-Scan In"=w287) -> ("Averaged BScan"=w286:dbl[])  [unwired: 10 in]
              n133 = call "OCT Processing 2ch functional global.vi"("State"=processing_states."Set Background", "Background"=w286) -> ()  [unwired: 9 in, 5 out]
            }
          }
        }
        n134 = Enqueue Element(queue=w256, element=OCT_Hardware_States."Set Resampling Array", error in (no error)=w259) -> ()  [unwired: 1 in, 3 out]
      }
      frame "Aquire and Save" {
        # "Close files and set save \nstate to do nothing"
        # "Update and \nclear the \nEn Face"
        # "Tell the FFT the most\nup-to-date imaging\nparameters"
        n135 = local read "Imaging Parameters"() -> (w323:T4)
        n136 = call "galvo_functional_global.vi"("State"=galvo_states."Run Raster", "error in (no error)"=w311) -> ("error out"=w308:errorcluster)  [unwired: 8 in, 1 out]
        n137 = call <vilib>:"Clear Errors.vi"("error in (no error)"=w308) -> ("error out"=w328:errorcluster)  [unwired: 5 in, 1 out]
        n138 = call "OCT Processing 2ch functional global.vi"("State"=processing_states."Update Imaging Parameters", "Input Parameters"=w323, "error in (no error)"=w328) -> ("error out"=w297:errorcluster)  [unwired: 8 in, 4 out]
        n139 = call "Save Data Functional Global.vi"("States"=Saving_Data_States."Get Queue", "error in (no error)"=w328) -> ("error out"=w299:errorcluster, "Saving Queue Out"=w314:refnum<queue>)  [unwired: 6 in, 2 out]
        n140 = call "galvo_functional_global.vi"("State"=galvo_states."Get Scan Parameters", "error in (no error)"=w297) -> ("error out"=w298:errorcluster, "Scanning Output"=w309:T27)  [unwired: 8 in]
        n141 = local read "Async_Setting"() -> (w302:T5)
        n142 = local read "Data Format"() -> (w303:T1)
        n143 = call "En Face Functional Global.vi"("En Face States"=En_Face_States."Clear En Face", "Error In"=w298, "Scanning"=w309) -> ("Error Out"=w296:errorcluster)  [unwired: 8 in]
        n144 = call "Quick NPT Config.vi"("error in (no error)"=w299, "Data Format"=w303, "Async_Setting"=w302, "Value"=w300) -> ("error out"=w295:errorcluster, "Device Out"=w301:i32)  [unwired: 4 in, 1 out]
        n145 = Merge Errors(w295, w296) -> (w294:errorcluster)
        n146 = call "OCT Processing 2ch functional global.vi"("State"=processing_states."Get Queue", "error in (no error)"=w294) -> ("queue out"=w316:refnum<queue>, "error out"=w318:errorcluster)  [unwired: 9 in, 3 out]
        n147 = while {
          tunnel: w318 -> [_]
          tunnel: [w334] -> w305
          i -> [w333]
          stop <- w332 stop-if-true
          # "Saves data as long as data is being fed into the Queue,\notherwise it will time out and halt this loop."
          n148 = case shown="1, Default" w333 {
            tunnel: [FALSE w337] -> w332
            tunnel: [_ w338] -> w334
            frame 0 {
              # "Wait for data to Q up"
              n149 = Wait (ms)(milliseconds to wait=u32 500) -> ()  [unwired: 1 out]
            }
            frame 1, Default {
              n150 = local read "Data Format"() -> (w340:T1)
              n151 = Wait (ms)(milliseconds to wait=u32 10) -> ()  [unwired: 1 out]
              n152 = call "Save Data Functional Global.vi"("States"=Saving_Data_States."Save Data", "Data Format"=w340) -> ("error out"=w338:errorcluster, "Time Out"=w337:bool)  [unwired: 6 in, 2 out]
            }
          }
        }
        n153 = while {
          shift-right: [ATS_Async_Ctrl."Get" ("ATS_Async_Ctrl")] -> _
          shift-left: ATS_Async_Ctrl."StartCapture" ("ATS_Async_Ctrl") -> [w353]
          tunnel: w316 -> [w349]
          tunnel: w314 -> [w348]
          tunnel: w301 -> [w343]
          stop <- w347 stop-if-true
          n154 = call "ATS_AsyncDMA_Device.vi"("DeviceIn"=w343, "ATS_Async_Ctrl"=w353) -> ("Buffer"=w351:u16[], "Async_Status"=w346:T36)  [unwired: 9 in, 3 out]
          n155 = local read "Reset DAQ"() -> (w350:bool)
          n156 = call "DAQ Status.vi"("Enum"=DAQ_Status_States."Get", "Async_Status"=w346) -> ("DAQ Error?"=w344:bool, "Valid"=w345:bool)  [unwired: 8 in]
          n157 = Compound Arithmetic op=OR(w344, w350) -> (w347:bool)
          n158 = case shown="True" w345 {
            tunnel: w351 -> [_ w356]
            tunnel: w351 -> [_ w357]
            tunnel: w349 -> [_ w358]
            tunnel: w348 -> [_ w355]
            frame False {
              # "Do nothing"
            }
            frame True {
              w354 = 50 ("timeout in ms (-1)")
              n159 = Enqueue Element(queue=w355, element=w356, timeout in ms (-1)=w354) -> ()  [unwired: 1 in, 3 out]
              n160 = Enqueue Element(queue=w358, element=w357, timeout in ms (-1)=w354) -> ()  [unwired: 1 in, 3 out]
            }
          }
        }
        n161 = while {
          tunnel: [w330] -> w304
          tunnel: w305 -> [w330]
          stop <- w329 stop-if-true
          n162 = local read "Processing Finished"() -> (w329:bool)
          n163 = Wait (ms)(milliseconds to wait=u32 25) -> ()  [unwired: 1 out]
        }
        n164 = call "galvo_functional_global.vi"("State"=galvo_states."Reset", "error in (no error)"=w304) -> ("error out"=w307:errorcluster)  [unwired: 8 in, 1 out]
        n165 = call "Save Data Functional Global.vi"("States"=Saving_Data_States."Close Files", "error in (no error)"=w307) -> ("error out"=w322:errorcluster)  [unwired: 6 in, 3 out]
        n166 = call "Save Data Functional Global.vi"("States"=Saving_Data_States."Do Nothing" ("Save State"), "error in (no error)"=w322) -> ("error out"=w320:errorcluster)  [unwired: 6 in, 3 out]
        n167 = Enqueue Element(queue=w325, element=OCT_Hardware_States."Acquire Data", error in (no error)=w320) -> ()  [unwired: 1 in, 3 out]
      }
      frame "Wait" {
        n168 = Wait (ms)(milliseconds to wait=u32 10) -> ()  [unwired: 1 out]
      }
      frame "Stop" {
        n169 = Release Queue(queue=w370, error in (no error)=w369) -> (error out=w368:errorcluster)  [unwired: 1 in, 2 out]
        n170 = call "OCT Processing 2ch functional global.vi"("State"=processing_states."Shutdown", "error in (no error)"=w368) -> ("error out"=w367:errorcluster)  [unwired: 9 in, 4 out]
        n171 = call "Save Data Functional Global.vi"("States"=Saving_Data_States."Shutdown", "error in (no error)"=w367) -> ("error out"=w364:errorcluster)  [unwired: 6 in, 3 out]
        n172 = call "galvo_functional_global.vi"("State"=galvo_states."Shutdown", "error in (no error)"=w364) -> ("error out"=w363:errorcluster)  [unwired: 8 in, 1 out]
        n173 = flat-sequence {
          tunnel: w363 -> [_]
          frame #0 {
            w374 = 0 ("DeviceIn")
            n174 = call "ATS_AsyncDMA_Device.vi"("DeviceIn"=w374, "ATS_Async_Ctrl"=ATS_Async_Ctrl."Stop") -> ("ReadSamples_Out"=w373:T30)  [unwired: 9 in, 4 out]
            n175 = call "ATS_AsyncDMA_Device.vi"("DeviceIn"=w374, "ATS_Async_Ctrl"=ATS_Async_Ctrl."Abort", "ReadSamples"=w373) -> ()  [unwired: 8 in, 5 out]
          }
          frame #1 {
            n176 = Stop(stop? (T)=TRUE) -> ()
          }
        }
      }
      frame "Initialize Clock" {
        w379 = T15 12 items=["20mV", "40mV", "50mV", "80mV", "100mV", "200mV", "400mV", "500mV", "800mV", "1 V", "1.25 V", "2 V", "4 V", "5 V", "8 V", "10 V", "16 V", "20 V", "40 V", "HiFi"] ("Input B.Range")
        w382 = u32 18 items=["1 kS/s", "2 kS/s", "5 kS/s", "10 kS/s", "20 kS/s", "50 kS/s", "100 kS/s", "200 kS/s", "500 kS/s", "1 MS/s", "2 MS/s", "5 MS/s", "10 MS/s", "20 MS/s", "50 MS/s", "100 MS/s", "125 MS/s", "160 MS/s", "180 MS/s"] ("ClckRate")
        n177 = local read "Clock Length"() -> (w381:u32)
        n178 = call "ATS_Device.vi"("BoardToVerify"=w377, "ATS_Check"=ATS_Check_Ctrl."Verify Board", "DevCtrl"=Device_Ctrl."Initialize", "DeviceIn"=0 ("Device")) -> ("error out"=w384:errorcluster, "DeviceOut"=w389:i32)  [unwired: 1 in, 5 out]
        n179 = Bundle By Name(cluster=w376, "Record.Length"=w381, "Clock.ClckSource"=ClockSource."Internal", "Clock.ClckRate"=w382, "Input B.Range"=w379, "Input A.Impedance"=Impedance."50 ohms") -> (w380:T7)
        n180 = call "ATS_Device.vi"("error in (no error)"=w384, "DevCtrl"=Device_Ctrl."Abort", "DeviceIn"=w389) -> ("DeviceOut"=w387:i32)  [unwired: 2 in, 6 out]
        n181 = call "ATS_MS_Set_Device.vi"("Set_Manually (F)"=FALSE, "Setup_In"=w380, "DeviceIn"=w387) -> ()  [unwired: 3 in, 6 out]
      }
      frame "Set Resampling Array" {
      }
      frame "Update DAQ Parameters" {
        n182 = call "Configure Alazar Cluster.vi"("Alazar Board"=w393) -> ("Output Reference"=w395:refnum<vi>)  [unwired: 10 in]
        n183 = property class="Clust (strict)"(reference=w395) -> ("Value"=w394:T7)  [unwired: 1 in, 2 out]
      }
      frame "K-Space Calibration" {
        n184 = Enqueue Element(queue=w408, element=OCT_Hardware_States."Update DAQ Parameters", error in (no error)=w407) -> (queue out=w396:refnum<queue>, error out=w405:errorcluster)  [unwired: 1 in, 1 out]
        n185 = call "Display Message to User"("error in (no error)"=w405) -> ("error out"=w398:errorcluster)  [unwired: 9 in, 1 out]
        n186 = call "galvo_functional_global.vi"("State"=galvo_states."Center Galvos", "error in (no error)"=w398) -> ("error out"=w397:errorcluster)  [unwired: 8 in, 1 out]
        n187 = Enqueue Element(queue=w396, element=OCT_Hardware_States."Set Resampling Array", error in (no error)=w397) -> (error out=w399:errorcluster)  [unwired: 1 in, 2 out]
        n188 = property on="Calibrate" class="Bool"(error in=w399, "Visible"=TRUE) -> (error out=w401:errorcluster)  [unwired: 1 in, 1 out]
        n189 = property on="Calibrate" class="Bool"(error in=w401, "Blinking"=TRUE) -> ()  [unwired: 1 in, 2 out]
      }
      frame "Background Subtraction" {
        n190 = call "Display Message to User2"("error in (no error)"=w415) -> ("error out"=w416:errorcluster)  [unwired: 9 in, 1 out]
        n191 = call "galvo_functional_global.vi"("State"=galvo_states."Center Galvos", "error in (no error)"=w416) -> ("error out"=w411:errorcluster)  [unwired: 8 in, 1 out]
        n192 = Enqueue Element(queue=w413, element=OCT_Hardware_States."Initialize DAQ", error in (no error)=w411) -> (queue out=w412:refnum<queue>, error out=w410:errorcluster)  [unwired: 1 in, 1 out]
        n193 = Enqueue Element(queue=w412, element=OCT_Hardware_States."Acquire Background", error in (no error)=w410) -> ()  [unwired: 1 in, 3 out]
      }
      frame "Allocate OpenCL Memory" {
      }
      frame "Delete OpenCL Memory" {
      }
    }
  }
  n194 = while {
    tunnel: w9 -> [w422]
    tunnel: w10 -> [w423]
    stop <- FALSE stop-if-true
    # "User Interface Loop"
    n195 = event shown="[4] Menu Selection (User)" {
      selector: w423 -> [_ _ _ _ _ _ _]
      dyn-events: _ -> [_ _ _ _ _ _ _]
      timeout: _ -> [_ _ _ _ _ _ _]
      tunnel: w422 -> [w425 w429 w439 _ w453 _ _]
      event User Event {
        n196 = event-data() -> ("Reset Galvos"=w427:bool)  [unwired: 1 in]
        n197 = local write "Reset DAQ"(w427) -> ()
        n198 = Enqueue Element(queue=w425, element=OCT_Hardware_States."Initialize DAQ") -> ()  [unwired: 2 in, 3 out]
      }
      event "Stop Button": Value Change {
        n199 = event-data() -> ()  [unwired: 1 in, 1 out]
        n200 = flat-sequence {
          tunnel: w429 -> [w433]
          tunnel: [w433] -> w430
          tunnel: [50] -> w428
          tunnel: w430 -> [w435]
          tunnel: w428 -> [w434]
          frame #0 {
            w432 = TRUE ("Reset DAQ")
            n201 = local write "Processing Finished"(w432) -> ()
            n202 = local write "Reset DAQ"(w432) -> ()
          }
          frame #1 {
            n203 = Wait (ms)(milliseconds to wait=w434) -> ()  [unwired: 1 out]
            n204 = Enqueue Element(queue=w435, element=OCT_Hardware_States."Stop") -> ()  [unwired: 2 in, 3 out]
          }
        }
      }
      event "Save Sweep": Value Change {
        n205 = event-data() -> ()  [unwired: 1 in, 1 out]
        n206 = flat-sequence {
          tunnel: [w440] -> w438
          tunnel: w438 -> [w446]
          tunnel: [w444] -> w437
          tunnel: w439 -> [w448]
          tunnel: w437 -> [_]
          frame #0 {
            n207 = call "File Dialog2"("prompt"="Select Path for saving") -> ("selected path"=w440:path)  [unwired: 11 in, 3 out]
          }
          frame #1 {
            n208 = local read "Imaging Parameters"() -> (w443:T4)
            n209 = local write "Save Data"(TRUE ("Save Data")) -> ()
            n210 = call "Save Data Functional Global.vi"("Input Parameters"=w443, "States"=Saving_Data_States."Create Files", "Folder"=w446) -> ("error out"=w444:errorcluster)  [unwired: 5 in, 3 out]
          }
          frame #2 {
            n211 = Enqueue Element(queue=w448, element=OCT_Hardware_States."Aquire and Save") -> ()  [unwired: 2 in, 3 out]
          }
          frame #3 {
            n212 = local write "Reset DAQ"(TRUE ("Reset DAQ")) -> ()
          }
        }
      }
      event User Event {
        n213 = event-data() -> ()  [unwired: 1 in, 1 out]
        n214 = call "OCT Processing 2ch functional global.vi"("State"=processing_states."Get Size") -> ("# elements in queue"=w451:i32)  [unwired: 10 in, 4 out]
        n215 = Equal To 0?(x=w451) -> (x = 0?=→"Processing Finished":bool)
      }
      event Menu Selection (User) {
        n216 = event-data() -> ("ItemTag"=w454:string)  [unwired: 1 in, 2 out]
        n217 = case shown="\"DAQ Status\"" w454 {
          tunnel: w453 -> [_ _ w458 _ _ w470 w474 _]
          frame "Raw Data", Default {
            n218 = call "Display Raw Data.vi"("Enum"=Display_Raw_Data_states."Show") -> ()  [unwired: 11 in]
          }
          frame "DAQ Status" {
            n219 = call "DAQ Status.vi"("Enum"=DAQ_Status_States."Show") -> ()  [unwired: 9 in, 2 out]
          }
          frame "Configure_DAQ" {
            n220 = flat-sequence {
              tunnel: w458 -> [w464]
              tunnel: [w464] -> w457
              frame #0 {
                n221 = local write "Reset DAQ"(TRUE ("Reset DAQ")) -> ()
              }
            }
            n222 = Enqueue Element(queue=w457, element=OCT_Hardware_States."Update DAQ Parameters") -> (queue out=w460:refnum<queue>, error out=w461:errorcluster)  [unwired: 2 in, 1 out]
            n223 = Enqueue Element(queue=w460, element=OCT_Hardware_States."Initialize DAQ", error in (no error)=w461) -> ()  [unwired: 1 in, 3 out]
          }
          frame "En Face" {
            n224 = call "En Face Functional Global.vi"("En Face States"=En_Face_States."Show") -> ()  [unwired: 10 in, 1 out]
          }
          frame "Save Sweep" {
            n225 = property on="Save Sweep" class="Bool (strict)"("Val(Sgnl)"=TRUE ("Value (Signaling)")) -> ()  [unwired: 2 in, 2 out]
          }
          frame "K-Space Correction" {
            n226 = Enqueue Element(queue=w470, element=OCT_Hardware_States."K-Space Calibration") -> (error out=w468:errorcluster)  [unwired: 2 in, 2 out]
            n227 = flat-sequence {
              tunnel: w468 -> [_]
              tunnel: [TRUE] -> w467
              frame #0 {
              }
            }
            n228 = local write "Reset DAQ"(w467) -> ()
          }
          frame "Background Subtraction" {
            n229 = Enqueue Element(queue=w474, element=OCT_Hardware_States."Background Subtraction") -> (error out=w473:errorcluster)  [unwired: 2 in, 2 out]
            n230 = flat-sequence {
              tunnel: [w477] -> _
              tunnel: w473 -> [w477]
              tunnel: [TRUE ("Reset DAQ")] -> w472
              frame #0 {
              }
            }
            n231 = local write "Reset DAQ"(w472) -> ()
          }
          frame "Configure_Galvos" {
            n232 = call "galvo_functional_global.vi"("State"=galvo_states."Show") -> ()  [unwired: 9 in, 2 out]
          }
        }
      }
      event "Save Sweep Button": Value Change {
        n233 = event-data() -> ()  [unwired: 1 in, 1 out]
        n234 = property on="Save Sweep" class="Bool (strict)"("Val(Sgnl)"=TRUE ("Value (Signaling)")) -> ()  [unwired: 2 in, 2 out]
      }
      event "Calibrate": Value Change {
        n235 = event-data() -> ()  [unwired: 1 in, 1 out]
        n236 = property on="Calibrate" class="Bool"("Visible"=FALSE) -> (error out=w484:errorcluster)  [unwired: 2 in, 1 out]
        n237 = property on="Calibrate" class="Bool"(error in=w484, "Blinking"=FALSE) -> ()  [unwired: 1 in, 2 out]
        n238 = call "Display Raw Data.vi"("Enum"=Display_Raw_Data_states."Add Raw") -> ()  [unwired: 11 in]
        n239 = call "Clock Frequency generator hilbert without wavepond.vi"() -> ("Zero Crossing Resample Index"=w480:i32[])  [unwired: 11 in]
        n240 = call "OCT Processing 2ch functional global.vi"("State"=processing_states."Set Reample Array", "Resample Array"=w480) -> ()  [unwired: 9 in, 5 out]
      }
    }
  }
  n241 = while {
    stop <- w493 stop-if-true
    # "Display Loop"
    # "Sometimes a timeout event sends\na 0 array, this stops the flickering\nof the front panl due to those \ntimeout events"
    # "This takes the 0th element of the processed data,\nthe other elements will NOT be displayed"
    # "This loop just gets the last b-scan processed wheter in real time mode or not. \nJust meant to update the front panel Asynchronously.  This frame is NOT\nguarenteed to view every BScan, just the last one processed."
    n242 = call "OCT Processing 2ch functional global.vi"("State"=processing_states."Get Last Processed BScan") -> ("Processed OCT Data"=w490:T28)  [unwired: 10 in, 4 out]
    n243 = case shown="\"Channel A\", Default" "Display" {
      tunnel: w490 -> [w498 w499]
      tunnel: [w496 w500] -> w488
      frame "Channel A", Default {
        n244 = Unbundle By Name(w498) -> ("Intensity A"=w497:sgl[][][])
        n245 = Index Array(array=w497) -> (element=w496:sgl[][])  [unwired: 3 in]
      }
      frame "Channel B" {
        n246 = Unbundle By Name(w499) -> ("Intensity B"=w501:sgl[][][])
        n247 = Index Array(array=w501) -> (element=w500:sgl[][])  [unwired: 3 in]
      }
    }
    n248 = Array Size(array=w488) -> (size(s)=w489:i32[])
    n249 = Multiply Array Elements(1:w489) -> (0:w487:i32)
    n250 = Equal To 0?(x=w487) -> (x = 0?=w486:bool)
    n251 = case shown="False" w486 {
      tunnel: w488 -> [w494 _]
      frame False {
        "BScan" <- w494
      }
      frame True {
        n252 = Wait Until Next ms Multiple(millisecond multiple=u32 10) -> ()  [unwired: 1 out]
      }
    }
    n253 = local read "Stop Button"() -> (w493:bool)
  }
